vi "Home motors.vi"(4 "error in (no error)":errorcluster, 7 "Controller Reference In":refnum<k7>) -> (0 "error out":errorcluster, 3 "Controller Reference Out":refnum<k7>)   [LabVIEW 2015]
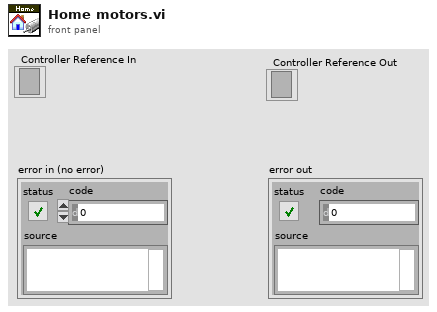
[diagram p1: front panel]
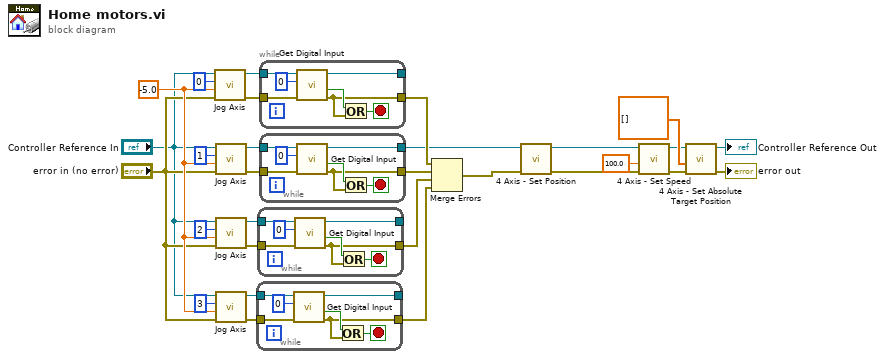
[diagram p0: block diagram]
diagram:
  w17 = sgl -5.0 ("Jog Speed")
  n1 = call "Jog Axis.vi"("error in (no error)"="error in (no error)", "Jog Speed"=w17, "Axis In"=i16 0, "Controller Reference"="Controller Reference In") -> ("error out"=w28:errorcluster, "Controller Reference out"=w29:refnum<k7>)  [unwired: 1 in, 1 out]
  n2 = call "Jog Axis.vi"("error in (no error)"="error in (no error)", "Jog Speed"=w17, "Axis In"=i16 1, "Controller Reference"="Controller Reference In") -> ("error out"=w26:errorcluster, "Controller Reference out"=w27:refnum<k7>)  [unwired: 1 in, 1 out]
  n3 = call "Jog Axis.vi"("error in (no error)"="error in (no error)", "Jog Speed"=w17, "Axis In"=i16 2, "Controller Reference"="Controller Reference In") -> ("error out"=w24:errorcluster, "Controller Reference out"=w25:refnum<k7>)  [unwired: 1 in, 1 out]
  n4 = call "Jog Axis.vi"("error in (no error)"="error in (no error)", "Jog Speed"=w17, "Axis In"=i16 3, "Controller Reference"="Controller Reference In") -> ("error out"=w22:errorcluster, "Controller Reference out"=w23:refnum<k7>)  [unwired: 1 in, 1 out]
  n5 = while {
    tunnel: w23 -> [w36]
    tunnel: w22 -> [w35]
    tunnel: [w32] -> w13
    tunnel: [w31] -> _
    stop <- w33 stop-if-true
    n6 = call "Get Digital Input.vi"("error in (no error)"=w35, "nInput"=i16 0, "Controller Reference"=w36) -> ("error out"=w32:errorcluster, "Boolean Value"=w34:bool, "Controller Reference out"=w31:refnum<k7>)  [unwired: 1 in, 1 out]
    n7 = Or(x=w34, y=w32) -> (x .or. y?=w33:bool)
  }
  n8 = while {
    tunnel: w25 -> [w43]
    tunnel: w24 -> [w42]
    tunnel: [w39] -> w14
    tunnel: [w38] -> _
    stop <- w40 stop-if-true
    n9 = call "Get Digital Input.vi"("error in (no error)"=w42, "nInput"=i16 0, "Controller Reference"=w43) -> ("error out"=w39:errorcluster, "Boolean Value"=w41:bool, "Controller Reference out"=w38:refnum<k7>)  [unwired: 1 in, 1 out]
    n10 = Or(x=w41, y=w39) -> (x .or. y?=w40:bool)
  }
  n11 = while {
    tunnel: w29 -> [w50]
    tunnel: w28 -> [w49]
    tunnel: [w46] -> w16
    tunnel: [w45] -> _
    stop <- w47 stop-if-true
    n12 = call "Get Digital Input.vi"("error in (no error)"=w49, "nInput"=i16 0, "Controller Reference"=w50) -> ("error out"=w46:errorcluster, "Boolean Value"=w48:bool, "Controller Reference out"=w45:refnum<k7>)  [unwired: 1 in, 1 out]
    n13 = Or(x=w48, y=w46) -> (x .or. y?=w47:bool)
  }
  n14 = while {
    tunnel: w27 -> [w57]
    tunnel: w26 -> [w56]
    tunnel: [w53] -> w15
    tunnel: [w52] -> w2
    stop <- w54 stop-if-true
    n15 = call "Get Digital Input.vi"("error in (no error)"=w56, "nInput"=i16 0, "Controller Reference"=w57) -> ("error out"=w53:errorcluster, "Boolean Value"=w55:bool, "Controller Reference out"=w52:refnum<k7>)  [unwired: 1 in, 1 out]
    n16 = Or(x=w55, y=w53) -> (x .or. y?=w54:bool)
  }
  n17 = Merge Errors(w16, w15, w14, w13) -> (w4:errorcluster)
  n18 = call "4 Axis - Set Position.vi"("error in (no error)"=w4, "Controller Reference In"=w2) -> ("error out"=w1:errorcluster, "Controller Reference Out"=w3:refnum<k7>)  [unwired: 4 in]
  n19 = call "4 Axis - Set Speed.vi"("error in (no error)"=w1, "Speed"=sgl 100.0, "Controller Reference In"=w3) -> ("error out"=w11:errorcluster, "Controller Reference Out"=w10:refnum<k7>)  [unwired: 3 in]
  n20 = call "4 Axis - Set Absolute Target Position.vi"("error in (no error)"=w11, "Positions"=sgl[] [], "Controller Reference In"=w10) -> ("error out"=→"error out":errorcluster, "Controller Reference Out"=→"Controller Reference Out":refnum<k7>)  [unwired: 3 in]
